vi "Relay_State.vi"(8 "error in (no error)":errorcluster, 10 "Relay_States":bool[](array[boolean]), 11 "USB-87Pn_Data In":T1) -> (0 "error out":errorcluster, 3 "USB-87Pn_Data Out":T1)   [LabVIEW 2019, in "USB-87P8_Manager.lvlib"]
uses:
  Module/USB-87P8_Manager.lvlib
  USB-87Pn_Data.ctl
  USB-87Pn.lvclass
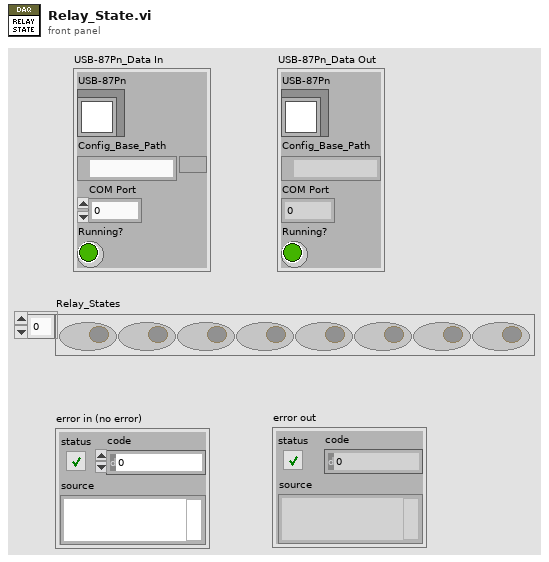
[diagram p1: front panel]
types:
  T1 = typedef "USB-87P8_Manager.lvlib/USB-87Pn_Data.ctl" = cluster{"USB-87Pn":refnum<class "USB-87Pn.lvclass">, "Config_Base_Path":path, "COM Port":i32, "Running?":bool}
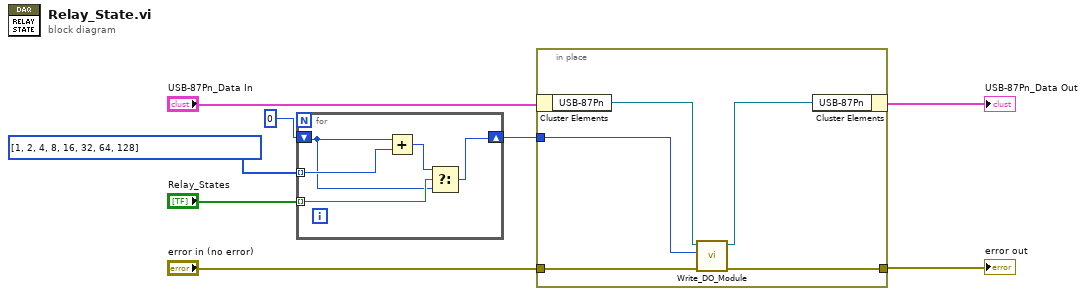
[diagram p0: block diagram]
diagram:
  n1 = for {
    tunnel: "Relay_States" -> [w13] mode=indexing
    tunnel: i32[] [1, 2, 4, 8, 16, 32, 64, 128] -> [w12] mode=indexing
    shift-right: [w9] -> w1
    shift-left: 0 -> [w10]
    n2 = Add(x=w10, y=w12) -> (x+y=w11:i32)
    n3 = Select(t=w11, s=w13, f=w10) -> (s? t:f=w9:i32)
  }
  n4 = in-place {
    in-place-border: "error in (no error)" -> [w16]
    in-place-border: [w15] -> w5
    in-place-border: w1 -> [w14]
    n5 = in-place-cluster #1("USB-87Pn_Data In") -> ("USB-87Pn"=w18:refnum<class "USB-87Pn.lvclass">)
    n6 = call "Write_DO_Module.vi"("error in (no error)"=w16, "DO_Value"=w14, "USB-87Pn in"=w18) -> ("error out"=w15:errorcluster, "USB-87Pn out"=w17:refnum<class "USB-87Pn.lvclass">)  [unwired: 7 in]
    n7 = in-place-cluster #1("USB-87Pn"=w17) -> (→"USB-87Pn_Data Out":T1)
  }
  "error out" <- w5
